vi "Write.vi"(8 "error in (no error)":errorcluster caption="错误输入（无错误）", 10 "buf":string, 11 "Serial 输入":refnum<class "Serial.lvclass"> caption="DNL_LabVIEW Object in") -> (0 "error out":errorcluster caption="错误输出", 3 "Serial 输出":refnum<class "Serial.lvclass"> caption="DNL_LabVIEW Object out")   [LabVIEW 2012, in "Serial.lvclass"]
uses:
  Serial.lvclass
  PComm/PCOMM.lvlib
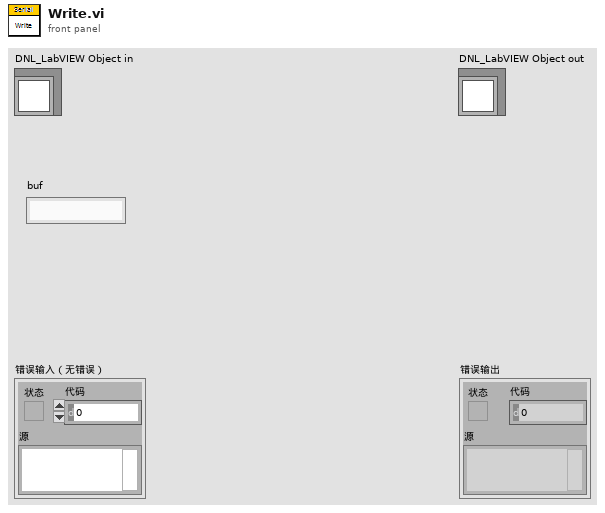
[diagram p1: front panel]
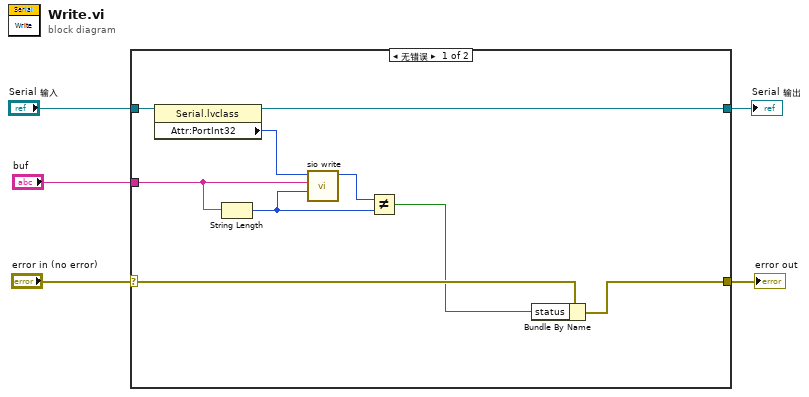
[diagram p0: block diagram]
diagram:
  n1 = case shown="无错误" "error in (no error)" {
    selector: "error in (no error)" -> [w10 w16]
    tunnel: [w9 w16] -> w4
    tunnel: [w11 w15] -> w2
    tunnel: "Serial 输入" -> [w14 w15]
    tunnel: "buf" -> [w12 _]
    frame No Error {
      n2 = property class="Serial.lvclass"(reference=w14) -> (reference out=w11:refnum<class "Serial.lvclass">, "Attr:PortInt32"=w13:i32)  [unwired: 1 in, 1 out]
      n3 = String Length(string=w12) -> (length=w8:i32)
      n4 = call "sio write.vi"("len"=w8, "buf"=w12, "port"=w13) -> ("function return"=w7:i32)  [unwired: 7 in, 1 out]
      n5 = Not Equal?(x=w7, y=w8) -> (x != y?=w6:bool)
      n6 = Bundle By Name(cluster=w10, "status"=w6) -> (w9:errorcluster)
    }
    frame Error {
    }
  }
  "error out" <- w4
  "Serial 输出" <- w2
